vi "LVDatasetTest.vi"() -> ()   [LabVIEW 2011]
uses:
  <vilib>/Utility/file.llb/Read From Spreadsheet File (DBL).vi
  TrackerVIs/TrackerDLL.vi
panel:
  out "XCor  X & Y error":cluster{dbl, dbl}(graph)
  out "COM X & Y error":cluster{dbl, dbl}(graph)
  out "subarray":dbl[][](array[numeric])
  out "text file path":path
  out "File":string caption="Result"
  in  "Image count":i32=1
  out "Image":T1(plugin-control)
  out "COM":cluster{"comX":sgl, "comY":sgl}
  out "xcorpos":cluster{"XCor X":sgl, "XCor Y":sgl}
  out "median":sgl
  out "debug":T1(plugin-control)
  out "X autocor":sgl[](graph)
  out "Y autocor":sgl[](graph)
  out "Y profile":sgl[](graph)
  out "X profile":sgl[](graph)
  in  "xcor_iterations":i32=1
  out "Radial profile":sgl[](graph)
  in  "Path":path=path "D:/jcnossen1/ztracker/Qpaper_007LUT_varyRoi80/tmp_002"
  in  "Browse?":bool=TRUE
  in  "debug library":bool=TRUE
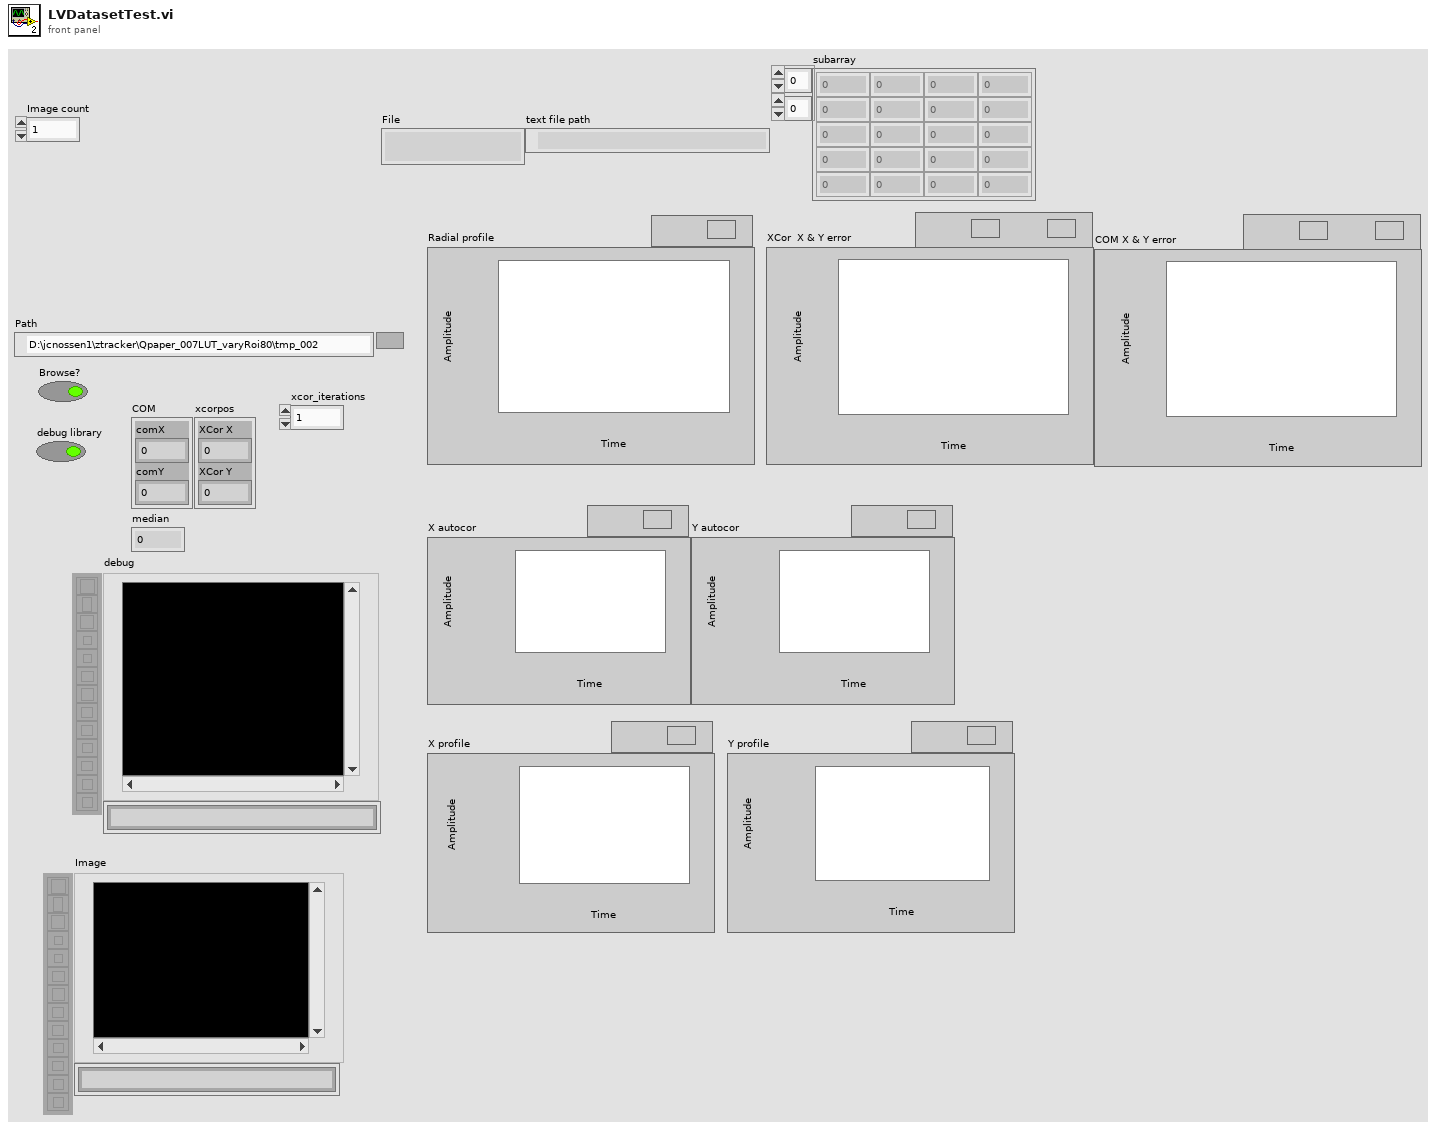
[diagram p1: front panel]
types:
  T1 = typedef "IMAQ Image.ctl" = refnum<image>
  T2 = typedef "Image Type" = u32
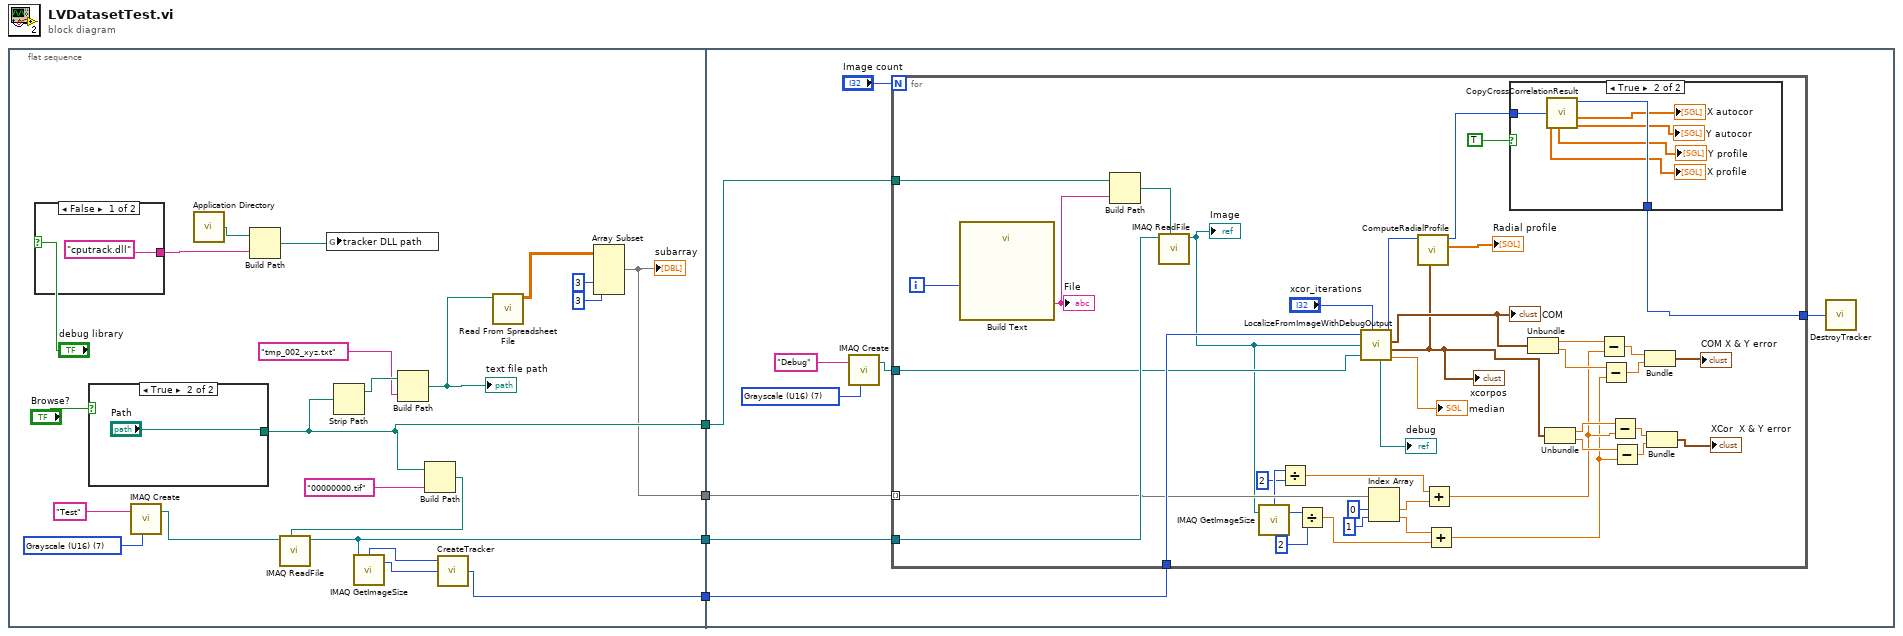
[diagram p0: block diagram]
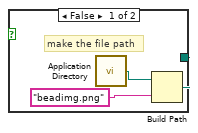
[diagram p2: hidden frame]
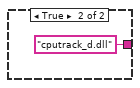
[diagram p3: hidden frame]
diagram:
  n1 = flat-sequence {
    tunnel: [w12] -> w4
    tunnel: [w14] -> w3
    tunnel: [w13] -> w2
    tunnel: [w5] -> w1
    tunnel: w4 -> [w40]
    tunnel: w3 -> [w39]
    tunnel: w2 -> [w38]
    tunnel: w1 -> [w33]
    frame #0 {
      w21 = T2 7 items=["Grayscale (U8)", "Grayscale (I16)", "Grayscale (SGL)", "Complex (CSG)", "RGB (U32)", "HSL (U32)", "RGB (U64)", "Grayscale (U16)"] ("Image Type")
      n2 = case shown="False" "debug library" {
        tunnel: ["cputrack.dll" "cputrack_d.dll"] -> w25
        frame False {
        }
        frame True {
        }
      }
      n3 = case shown="True" "Browse?" {
        tunnel: [w27 "Path"] -> w12
        frame False {
          # "make the file path"
          n4 = call <vilib>:"Application Directory.vi"() -> ("Application Directory"=w28:path)
          n5 = Build Path(base path=w28, name or relative path="beadimg.png") -> (appended path=w27:path)
        }
        frame True {
        }
      }
      n6 = call "IMAQ Create"("Image Name"="Test" ("String"), "Image Type"=w21) -> ("New Image"=w18:T1)  [unwired: 3 in, 1 out]
      n7 = call <vilib>:"Application Directory.vi"() -> ("Application Directory"=w24:path)
      n8 = Build Path(base path=w24, name or relative path=w25) -> (appended path=w26:path)
      n9 = global write "TrackerDLL.vi" "tracker DLL path"(w26) -> ()
      n10 = Strip Path(path=w12) -> (stripped path=w11:path)  [unwired: 1 out]
      n11 = Build Path(base path=w11, name or relative path="tmp_002_xyz.txt") -> (appended path=w9:path)
      "text file path" <- w9
      n12 = Build Path(base path=w12, name or relative path="00000000.tif") -> (appended path=w17:path)
      n13 = call "IMAQ ReadFile"("File Path"=w17, "Image"=w18) -> ("Image Out"=w13:T1)  [unwired: 5 in, 4 out]
      n14 = call "IMAQ GetImageSize"("Image"=w13) -> ("Y Resolution"=w15:i32, "X Resolution"=w16:i32)  [unwired: 3 in, 1 out]
      n15 = call "CreateTracker.vi"("height"=w15, "width"=w16) -> ("return type"=w14:u64)  [unwired: 1 in]
      n16 = call-poly <vilib>:"Read From Spreadsheet File.vi"("file path (dialog if empty)"=w9) -> ("all rows"=w8:dbl[][])  [unwired: 6 in, 4 out]
      n17 = Array Subset(array=w8, index (col)=3 ("index"), length (col)=3 ("length")) -> (w5:dbl[][])  [unwired: 2 in]
      "subarray" <- w5
    }
    frame #1 {
      w35 = T2 7 items=["Grayscale (U8)", "Grayscale (I16)", "Grayscale (SGL)", "Complex (CSG)", "RGB (U32)", "HSL (U32)", "RGB (U64)", "Grayscale (U16)"] ("Image Type")
      n18 = call "IMAQ Create"("Image Name"="Debug" ("String"), "Image Type"=w35) -> ("New Image"=w34:T1)  [unwired: 3 in, 1 out]
      n19 = for {
        N: "Image count" -> [_]
        tunnel: w40 -> [w74]
        tunnel: w39 -> [w72]
        tunnel: w38 -> [w70]
        tunnel: [w69] -> w37
        tunnel: w34 -> [w68]
        tunnel: w33 -> [w65] mode=indexing
        i -> [w71]
        n20 = call "Build Text"("ImageNumber"=w71) -> ("Result"=w75:string)  [unwired: 13 in, 1 out]
        "File" <- w75
        n21 = Build Path(base path=w74, name or relative path=w75) -> (appended path=w73:path)
        n22 = call "IMAQ ReadFile"("File Path"=w73, "Image"=w70) -> ("Image Out"=w48:T1)  [unwired: 5 in, 4 out]
        "Image" <- w48
        n23 = call "IMAQ GetImageSize"("Image"=w48) -> ("Y Resolution"=w44:i32, "X Resolution"=w47:i32)  [unwired: 3 in, 1 out]
        n24 = Divide(x=w47, y=2) -> (x/y=w45:dbl)
        n25 = Divide(x=w44, y=2) -> (x/y=w42:dbl)
        n26 = call "LocalizeFromImageWithDebugOutput.vi"("tracker"=w72, "xcor_iterations"="xcor_iterations", "input image"=w48, "debug image"=w68) -> ("tracker"=w80:u64, "COM"=w67:cluster{"X":sgl, "Y":sgl}, "debug image"=→"debug":T1, "xcorpos"=w66:cluster{"X":sgl, " Y":sgl}, "median"=→"median":sgl)  [unwired: 2 in]
        "COM" <- w67
        "xcorpos" <- w66
        n27 = Index Array(array=w65, index #1=0 ("index"), index #2=1 ("index")) -> (element #1=w52:dbl, element #2=w51:dbl)
        n28 = call "ComputeRadialProfile.vi"("center"=w66, "tracker"=w80) -> ("output"=→"Radial profile":sgl[], "tracker"=w81:u64)  [unwired: 8 in]
        n29 = Add(x=w45, y=w52) -> (x+y=w50:dbl)
        n30 = Add(x=w51, y=w42) -> (x+y=w49:dbl)
        n31 = case shown="True" TRUE {
          tunnel: w81 -> [w83 w84]
          tunnel: [w83 w89] -> w69
          frame False {
          }
          frame True {
            n32 = call "CopyCrossCorrelationResult.vi"("tracker"=w84) -> ("x prof"=→"X profile":sgl[], "y prof"=→"Y profile":sgl[], "tracker"=w89:u64, "x result"=→"X autocor":sgl[], "y_result"=→"Y autocor":sgl[])  [unwired: 3 in]
          }
        }
        n33 = Unbundle(w67) -> ("X"=w62:sgl, "Y"=w61:sgl)
        n34 = Unbundle(w66) -> ("X"=w57:sgl, "Y"=w56:sgl)
        n35 = Subtract(x=w62, y=w50) -> (x-y=w60:dbl)
        n36 = Subtract(x=w61, y=w49) -> (x-y=w59:dbl)
        n37 = Subtract(x=w57, y=w50) -> (x-y=w55:dbl)
        n38 = Subtract(x=w56, y=w49) -> (x-y=w54:dbl)
        n39 = Bundle(w60, w59) -> (→"COM X & Y error":cluster{dbl, dbl})  [unwired: 1 in]
        n40 = Bundle(w55, w54) -> (→"XCor  X & Y error":cluster{dbl, dbl})  [unwired: 1 in]
      }
      n41 = call "DestroyTracker.vi"("tracker"=w37) -> ()
    }
  }
